vi "calc_vswr.vi"(11 "abs":dbl) -> (3 "vswr":dbl)   [LabVIEW 2025]
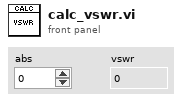
[diagram p1: front panel]
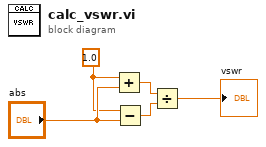
[diagram p0: block diagram]
diagram:
  w1 = 1.0 ("x")
  n1 = Add(x=w1, y="abs") -> (x+y=w3:dbl)
  n2 = Subtract(x=w1, y="abs") -> (x-y=w4:dbl)
  n3 = Divide(x=w3, y=w4) -> (x/y=→"vswr":dbl)
